vi "Reset beam staticstis.vi"(8 "error in (no error)":errorcluster, 11 "Beam in":refnum<class "Beam.lvclass">) -> (0 "error out":errorcluster, 3 "Beam out":refnum<class "Beam.lvclass">)   [LabVIEW 2019, in "Beam.lvclass"]
uses:
  Beam.lvclass
  Beam.lvclass/Beam.ctl
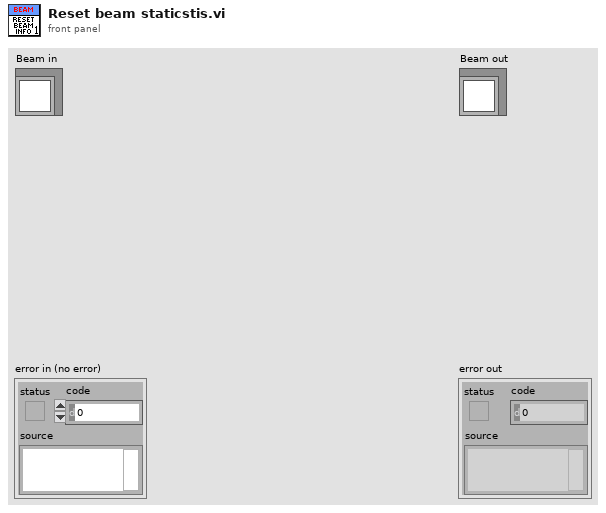
[diagram p1: front panel]
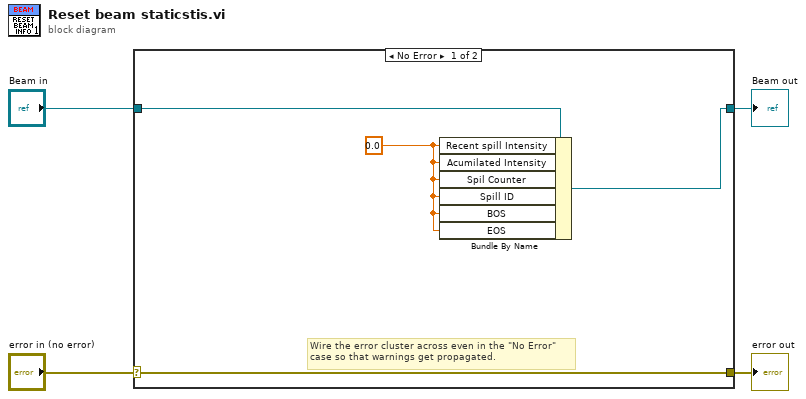
[diagram p0: block diagram]
diagram:
  n1 = case shown="No Error" "error in (no error)" {
    selector: "error in (no error)" -> [w8 w10]
    tunnel: [w8 w10] -> w3
    tunnel: [w6 w9] -> w1
    tunnel: "Beam in" -> [w7 w9]
    frame No Error {
      w5 = 0.0 ("Recent spill Intensity")
      # "Wire the error cluster across even in the \"No Error\"\ncase so that warnings get propagated."
      n2 = Bundle By Name(cluster=w7, "Recent spill Intensity"=w5, "Acumilated Intensity"=w5, "Spil Counter"=w5, "Spill ID"=w5, "BOS"=w5, "EOS"=w5) -> (w6:refnum<class "Beam.lvclass">)
    }
    frame Error {
    }
  }
  "error out" <- w3
  "Beam out" <- w1
